vi "UpdateFrameList.vi"(7 "Reverse":bool, 8 "error in (no error)":errorcluster, 9 "FlexRay:Timing Type":T1 items=["Cyclic", "Event", "Read"], 10 "XNET ECU":refnum<k21>, 11 "ListBox in":refnum<vi>) -> (0 "error out":errorcluster, 3 "Frames":refnum<k21>[](array[refnum]))   [LabVIEW 2020, in "FlexRay Custom Device System Explorer.lvlib"]
uses:
  FlexRay Custom Device System Explorer.lvlib
  Shared/FRFrameType.ctl
  <resource>/objmgr/xnet.rc
  Shared/FlexRay Custom Device Shared.lvlib
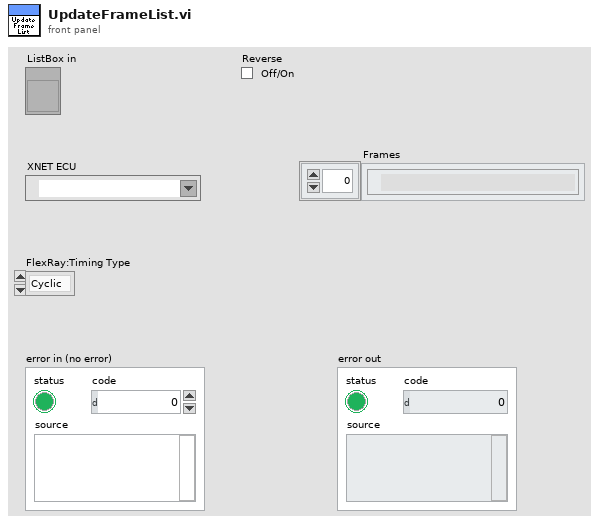
[diagram p1: front panel]
types:
  T1 = typedef "FlexRay Custom Device Shared.lvlib/FRFrameType.ctl" = u32
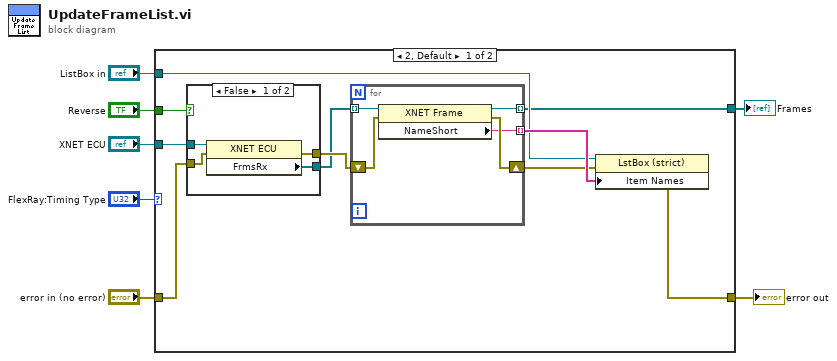
[diagram p0: block diagram]
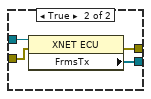
[diagram p2: hidden frame]
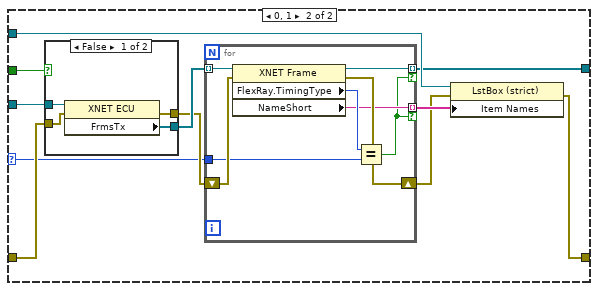
[diagram p3: hidden frame]
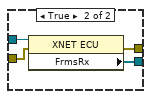
[diagram p4: hidden frame]
diagram:
  n1 = case shown="2, Default" "FlexRay:Timing Type" {
    selector: "FlexRay:Timing Type" -> [_ w34]
    tunnel: [w9 w32] -> w7
    tunnel: "error in (no error)" -> [w17 w41]
    tunnel: "XNET ECU" -> [w16 w38]
    tunnel: "Reverse" -> [w12 w37]
    tunnel: "ListBox in" -> [w11 w35]
    tunnel: [w8 w31] -> w1
    frame 2, Default {
      n2 = case shown="False" w12 {
        tunnel: w17 -> [w26 w30]
        tunnel: [w25 w29] -> w14
        tunnel: [w24 w28] -> w13
        tunnel: w16 -> [w23 w27]
        frame False {
          n3 = property class="XNET ECU"(reference=w23, error in=w26) -> (error out=w25:errorcluster, "FrmsRx"=w24:refnum<k21>[])  [unwired: 1 out]
        }
        frame True {
          n4 = property class="XNET ECU"(reference=w27, error in=w30) -> (error out=w29:errorcluster, "FrmsTx"=w28:refnum<k21>[])  [unwired: 1 out]
        }
      }
      n5 = for {
        shift-right: [w21] -> w10
        shift-left: w14 -> [w22]
        tunnel: w13 -> [w20] mode=indexing
        tunnel: [w19] -> w15 mode=indexing
        tunnel: [w18] -> w8 mode=indexing
        n6 = property class="XNET Frame"(reference=w20, error in=w22) -> (reference out=w18:refnum<k21>, error out=w21:errorcluster, "NameShort"=w19:string)
      }
      n7 = property on="Property Node" class="LstBox (strict)"(reference=w11, error in=w10, "Item Names"=w15) -> (error out=w9:errorcluster)  [unwired: 1 out]
    }
    frame 0, 1 {
      n8 = case shown="False" w37 {
        tunnel: w41 -> [w45 w49]
        tunnel: [w44 w48] -> w40
        tunnel: [w43 w47] -> w39
        tunnel: w38 -> [w42 w46]
        frame False {
          n9 = property class="XNET ECU"(reference=w42, error in=w45) -> (error out=w43:errorcluster, "FrmsTx"=w44:refnum<k21>[])  [unwired: 1 out]
        }
        frame True {
          n10 = property class="XNET ECU"(reference=w46, error in=w49) -> (error out=w47:errorcluster, "FrmsRx"=w48:refnum<k21>[])  [unwired: 1 out]
        }
      }
      n11 = for {
        tunnel: w34 -> [w55]
        shift-right: [w56] -> w33
        shift-left: w39 -> [w57]
        tunnel: w40 -> [w54] mode=indexing
        tunnel: [w52] -> w36 mode=indexing if=w50
        tunnel: [w51] -> w31 mode=indexing if=w50
        n12 = property class="XNET Frame"(reference=w54, error in=w57) -> (reference out=w51:refnum<k21>, error out=w56:errorcluster, "FlexRay.TimingType"=w53:u32, "NameShort"=w52:string)
        n13 = Equal?(x=w53, y=w55) -> (x = y?=w50:bool)
      }
      n14 = property on="Property Node" class="LstBox (strict)"(reference=w35, error in=w33, "Item Names"=w36) -> (error out=w32:errorcluster)  [unwired: 1 out]
    }
  }
  "error out" <- w7
  "Frames" <- w1
